vi "Load Theme-Root Only.vi"(8 "Error In":errorcluster, 10 "Theme File Path":path, 11 "Appearance Actor in":refnum<class "Appearance Actor.lvclass">) -> (0 "Error Out":errorcluster, 3 "Appearance Actor out":refnum<class "Appearance Actor.lvclass">)   [LabVIEW 2021, in "Appearance Actor.lvlib" / "Appearance Actor.lvclass"]
doc: "Load a theme from file using Theme Class.\n\n<B>This only has effect with Root Actor.</B>"
uses:
  Appearance Actor.lvclass
  C:/Program Files (x86)/National Instruments/LabVIEW 2021/vi.lib/ActorFramework/Actor/Actor.lvclass
  <vilib>/ActorFramework/Message Enqueuer/Message Enqueuer.lvclass
  <vilib>/ActorFramework/Actor/Actor.lvclass/Actor.ctl
  Appearance Actor.lvclass/Appearance Actor.ctl
  <vilib>/ActorFramework/Message Enqueuer/Message Enqueuer.lvclass/Message Enqueuer.ctl
  Appearance Actor Messages/Apply Theme Msg/Apply Theme Msg.lvclass/Apply Theme Msg.ctl
  <vilib>/ActorFramework/Message Enqueuer/Init from Existing Queue.vi
  <vilib>/ActorFramework/Message Enqueuer/Enqueue.vi
  Appearance Actor Messages/Propagate Theme To Nested Appearance Actors Msg/Propagate Theme To Nested Appearance Actors Msg.lvclass
  C:/Program Files (x86)/National Instruments/LabVIEW 2021/vi.lib/ActorFramework/Message/Message.lvclass
  Appearance Actor Messages/Apply Theme Msg/Apply Theme Msg.lvclass
  <vilib>/ActorFramework/Message Priority Queue/Priority Enqueue.vi
  Theme Classes/Generic Theme/Generic Theme.lvclass
  <vilib>/ActorFramework/Actor/Actor.lvclass
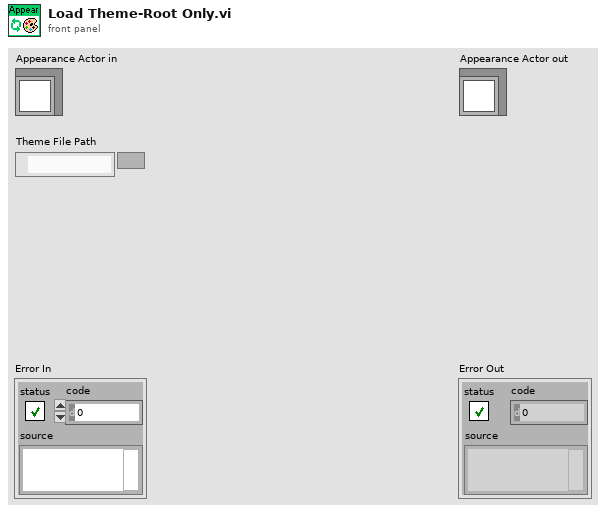
[diagram p1: front panel]
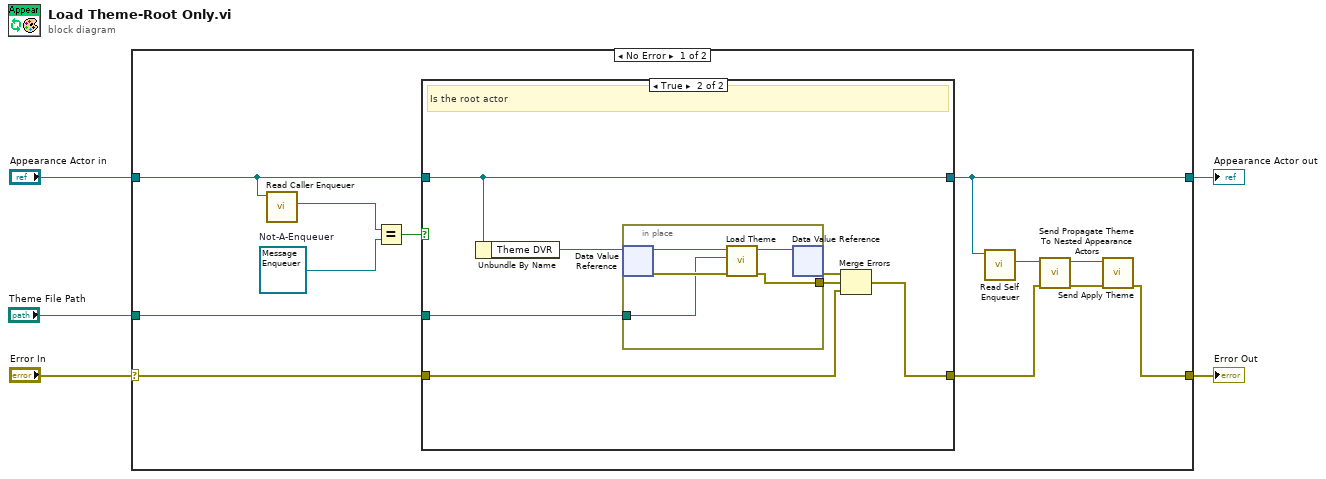
[diagram p0: block diagram]
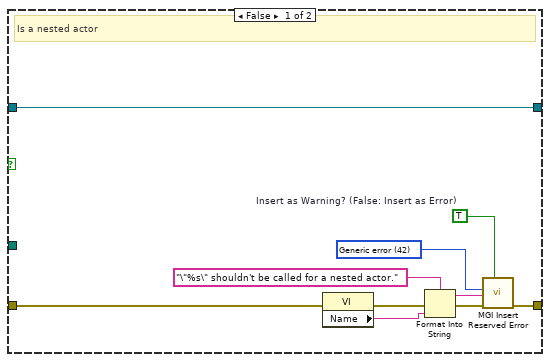
[diagram p2: hidden frame]
diagram:
  n1 = case shown="No Error" "Error In" {
    selector: "Error In" -> [w13 w41]
    tunnel: [w9 w41] -> w4
    tunnel: [w6 w40] -> w2
    tunnel: "Appearance Actor in" -> [w14 w40]
    tunnel: "Theme File Path" -> [w12 _]
    frame No Error {
      w16 = refnum<class "Message Enqueuer.lvclass"> refnum  # Not-A-Enqueuer
      n2 = call <vilib>:"Read Caller Enqueuer.vi"("Actor"=w14) -> ("Caller Enqueuer"=w17:refnum<class "Message Enqueuer.lvclass">)  [unwired: 10 in]
      n3 = Equal?(x=w17, y=w16) -> (x = y?=w15:bool)
      n4 = case shown="True" w15 {
        tunnel: w13 -> [w21 w28]
        tunnel: [w26 w29] -> w8
        tunnel: [w27 w34] -> w6
        tunnel: w14 -> [w27 w34]
        tunnel: w12 -> [_ w32]
        frame False {
          w24 = 42 items=["No error", "Argument error", "Memory is full", "Out of zone", "End of file", "File already open", "Generic file I/O error", "File not found", "File permission error", "Disk is full", "Duplicate path", "Too many files open", "System feature not enabled", "Resource file not found", "Cannot add resource", "Resource not found", "Image not found", "Image memory error", "Pen does not exist", "Config type invalid", "Config token not found", "Config parse error", "Config memory error", "Bad external code format", "Bad external code offset", "External code not present", "Null window", "Destroy window error", "Null menu", "Print aborted", "Bad print record", "Print driver error", "Windows error during printing", "Memory error during printing", "Print dialog error", "Generic print error", "Invalid device refnum", "Device not found", "Device parameter error", "Device unit error", "Cannot open device", "Device call aborted", "Generic error", "Cancelled by user", "Object ID too low", "Object ID too high", "Object not in heap", "Unknown heap", "Unknown object (invalid DefProc)", "Unknown object (DefProc not in table)", "Message out of range", "Invalid (null) method", "Unknown message", "Manager call not supported", "Bad address", "Network operation in progress", "Network operation timed out", "Connection is busy", "Network attribute not supported", "Network error", "Address in use", "System out of memory", "Connection aborted", "Connection refused", "Not connected", "Already connected", "Connection closed", "Initialization error (interapplication manager)", "Bad occurrence", "Wait on unbound occurrence handler", "Occurrence queue overflow", "Datalog type conflict", "Unused", "Unrecognized type (interapplication manager)", "Memory corrupt", "Failed to make temporary DLL", "Old CIN version", "Drag socket not found", "Failed to load drop-object", "Failed to register OLE object", "Failed to release OLE object", "Format specifier type mismatch", "Unknown format specifier", "Too few format specifiers", "Too many format specifiers", "Scan failed", "Newer CIN version", "OLE Convert", "Runtime menu error", "Password tampered", "Unknown error code"] ("Reserved Error Code (Generic error)")
          w25 = TRUE  # Insert as Warning? (False: Insert as Error)
          # "Is a nested actor"
          n5 = property class="VI"(error in=w21) -> (error out=w20:errorcluster, "Name"=w22:string)  [unwired: 1 in, 1 out]
          n6 = Format Into String(format string="\"%s\" shouldn't be called for a nested actor.", error in=w20, w22) -> (resulting string=w18:string, error out=w19:errorcluster)  [unwired: 1 in]
          n7 = call <userlib>:"MGI Insert Reserved Error.vi"("Insert as Warning? (False: Insert as Error)"=w25, "Error In"=w19, "Error Description"=w18, "Reserved Error Code (Generic error)"=w24) -> ("Error Out"=w26:errorcluster)  [unwired: 7 in]
        }
        frame True {
          # "Is the root actor"
          n8 = Unbundle By Name(w34) -> ("Theme DVR"=w33:refnum<data-value>)
          n9 = in-place {
            in-place-border: w32 -> [w37]
            in-place-border: [w35] -> w30
            n10 = in-place-dvr #1(w33) -> (w39:refnum<class "Generic Theme.lvclass">, w38:errorcluster)
            n11 = call-dynamic "Load Theme.vi"("Error In"=w38, "Theme File Path"=w37, "Generic Theme in"=w39) -> ("Error Out"=w35:errorcluster, "Generic Theme out"=w36:refnum<class "Generic Theme.lvclass">)  [unwired: 7 in]
            n12 = in-place-dvr #1(w36) -> (w31:errorcluster)  [unwired: 1 out]
          }
          n13 = Merge Errors(w31, w30, w28) -> (w29:errorcluster)
        }
      }
      n14 = call <vilib>:"Read Self Enqueuer.vi"("Actor"=w6) -> ("Self Enqueuer"=w7:refnum<class "Message Enqueuer.lvclass">)  [unwired: 10 in]
      n15 = call "Send Propagate Theme To Nested Appearance Actors.vi"("error in (no error)"=w8, "Message Enqueuer"=w7) -> ("error out"=w10:errorcluster, "Message Enqueuer out"=w11:refnum<class "Message Enqueuer.lvclass">)  [unwired: 8 in]
      n16 = call "Send Apply Theme.vi"("error in (no error)"=w10, "Message Enqueuer"=w11) -> ("error out"=w9:errorcluster)  [unwired: 8 in, 1 out]
    }
    frame Error {
    }
  }
  "Error Out" <- w4
  "Appearance Actor out" <- w2
